vi "FlatToRichnixnet_grpc_WaitRequest.vi"(5 "OutputClusterType":T1, 11 "InputCluster":T3) -> (3 "OutputCluster":T1)   [LabVIEW 2025, in "xnet-grpc_client.lvlib"]
uses:
  nixnet_grpc_WaitRequest_Flat.ctl
  nidevice_grpc_Session_Flat.ctl
  nixnet_grpc_WaitCondition.ctl
  nixnet_grpc_WaitRequest.ctl
  nixnet_grpc_WaitRequest_condition_enum/nixnet_grpc_WaitRequest_condition_enum.lvclass
  nidevice_grpc_Session.ctl
  xnet-grpc_client.lvlib
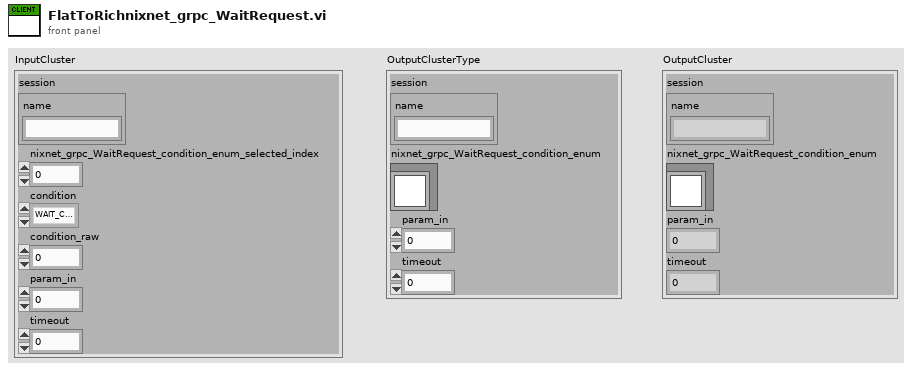
[diagram p1: front panel]
types:
  T1 = typedef "xnet-grpc_client.lvlib/nixnet_grpc_WaitRequest.ctl" = cluster{"session":T2, "nixnet_grpc_WaitRequest_condition_enum":refnum<class "nixnet_grpc_WaitRequest_condition_enum.lvclass">, "param_in":u32, "timeout":dbl}
  T2 = typedef "xnet-grpc_client.lvlib/nidevice_grpc_Session.ctl" = cluster{"name":string}
  T3 = typedef "xnet-grpc_client.lvlib/nixnet_grpc_WaitRequest_Flat.ctl" = cluster{"session":T4, "nixnet_grpc_WaitRequest_condition_enum_selected_index":i32, "condition":T5, "condition_raw":u32, "param_in":u32, "timeout":dbl}
  T4 = typedef "xnet-grpc_client.lvlib/nidevice_grpc_Session_Flat.ctl" = cluster{"name":string}
  T5 = typedef "xnet-grpc_client.lvlib/nixnet_grpc_WaitCondition.ctl" = enum32{"WAIT_CONDITION_UNSPECIFIED", "WAIT_CONDITION_TRANSMIT_COMPLETE", "WAIT_CONDITION_INTF_COMMUNICATING", "WAIT_CONDITION_INTF_REMOTE_WAKEUP", "WAIT_CONDITION_ETHERNET_SYNCED"}
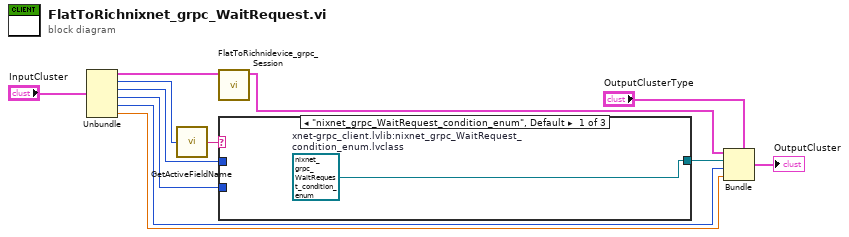
[diagram p0: block diagram]
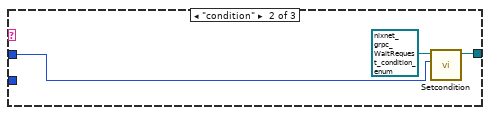
[diagram p2: hidden frame]
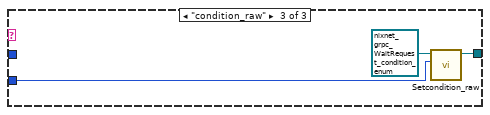
[diagram p3: hidden frame]
diagram:
  n1 = Unbundle "Unbundle"("InputCluster") -> ("session"=w9:T4, "nixnet_grpc_WaitRequest_condition_enum_selected_index"=w7:i32, "condition"=w4:T5, "condition_raw"=w3:u32, "param_in"=w2:u32, "timeout"=w1:dbl)
  n2 = call "GetActiveFieldName.vi"("protobuf index"=w7) -> ("oneof field name"=w6:string)
  n3 = call "FlatToRichnidevice_grpc_Session.vi"("InputCluster"=w9) -> ("OutputCluster"=w8:T2)  [unwired: 10 in]
  n4 = case "nixnet_grpc_WaitRequest_condition_enum" shown="\"nixnet_grpc_WaitRequest_condition_enum\", Default" w6 {
    tunnel: [w13 w15 w18] -> w5
    tunnel: w4 -> [_ w16 _]
    tunnel: w3 -> [_ _ w19]
    frame "nixnet_grpc_WaitRequest_condition_enum", Default {
      w13 = refnum<class "nixnet_grpc_WaitRequest_condition_enum.lvclass"> refnum  # xnet-grpc_client.lvlib:nixnet_grpc_WaitRequest_condition_enum.lvclass
    }
    frame "condition" {
      n5 = call "Setcondition.vi"("Set_Val"=w16, "OneOfTemplate in"=refnum<class "nixnet_grpc_WaitRequest_condition_enum.lvclass"> refnum) -> ("OneOfTemplate out"=w15:refnum<class "nixnet_grpc_WaitRequest_condition_enum.lvclass">)  [unwired: 8 in, 1 out]
    }
    frame "condition_raw" {
      n6 = call "Setcondition_raw.vi"("Set_Val"=w19, "OneOfTemplate in"=refnum<class "nixnet_grpc_WaitRequest_condition_enum.lvclass"> refnum) -> ("OneOfTemplate out"=w18:refnum<class "nixnet_grpc_WaitRequest_condition_enum.lvclass">)  [unwired: 8 in, 1 out]
    }
  }
  n7 = Bundle "Bundle"(cluster="OutputClusterType", "session"=w8, "nixnet_grpc_WaitRequest_condition_enum"=w5, "param_in"=w2, "timeout"=w1) -> (→"OutputCluster":T1)
